vi "udpLoop.vi"(8 "error in (no error)":errorcluster) -> (0 "error out":errorcluster)   [LabVIEW 2015]
uses:
  Shared Libraries/CustomVIs/CustomVI.lvlib
panel:
  out "Connections Attempted":i32
  out "Remote Port":u16
  out "Remote Address":string
  in  "Local Interface":string="10.10.20.1"
  in  "Local Port":u16=50000
  out "IMUvalues":dbl[](array[numeric])
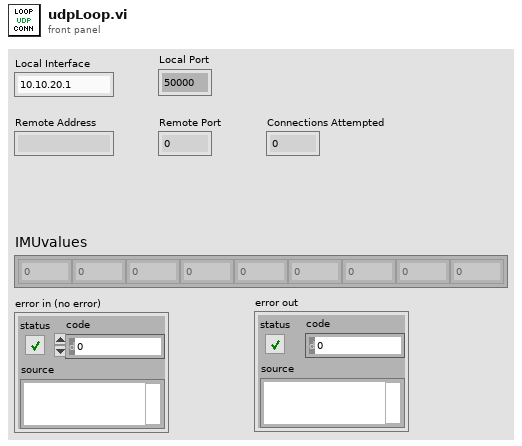
[diagram p1: front panel]
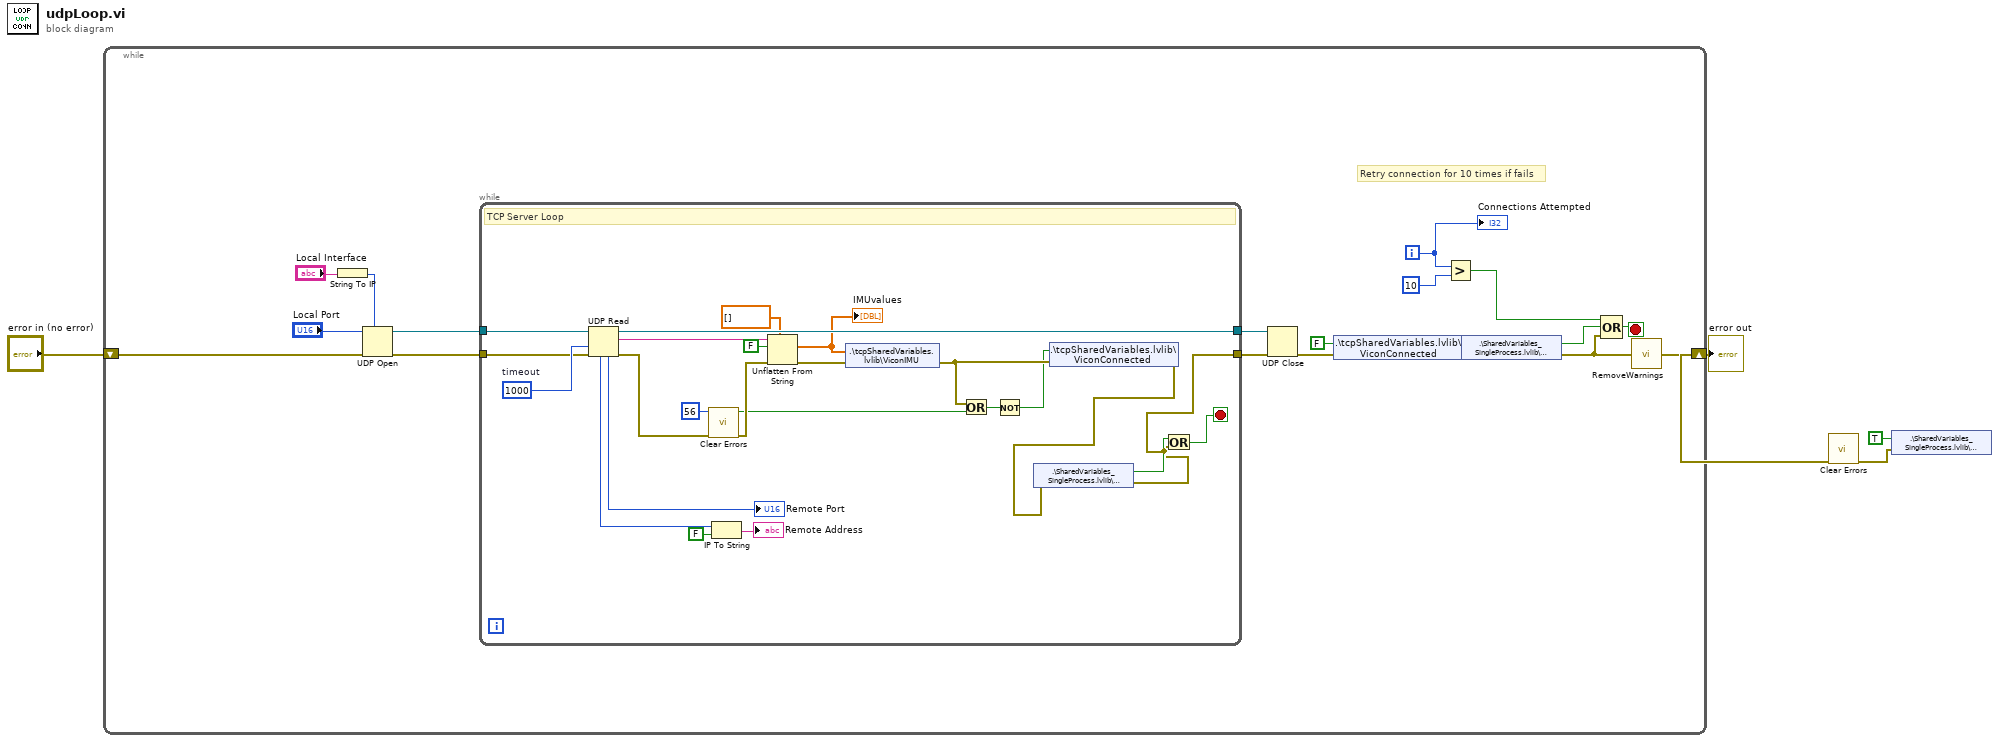
[diagram p0: block diagram]
diagram:
  n1 = while {
    shift-right: [w5] -> w1
    shift-left: "error in (no error)" -> [w17]
    i -> [w9]
    stop <- w14 stop-if-true
    # "Retry connection for 10 times if fails"
    n2 = String To IP(1:"Local Interface") -> (0:w21:u32)
    n3 = UDP Open(7:w21, 8:w17, 11:"Local Port") -> (port=w12:refnum<k16>, 0:w11:errorcluster)  [unwired: 2 in, 1 out]
    n4 = while {
      tunnel: [w27] -> w22
      tunnel: [w46] -> w10
      tunnel: w12 -> [w44]
      tunnel: w11 -> [w43]
      stop <- w28 stop-if-true
      w45 = 1000  # timeout
      # "TCP Server Loop"
      n5 = UDP Read(connection ID=w44, timeout ms (25000)=w45, 8:w43) -> (data out=w42:string, error out=w33:errorcluster, 3:w46:refnum<k16>, 4:→"Remote Port":u16, 6:w38:u32)  [unwired: 1 in]
      n6 = call <vilib>:"Clear Errors.vi"("error in (no error)"=w33, "specific error code to clear (0: all)"=56) -> ("error out"=w31:errorcluster, "specific error cleared?"=w26:bool)  [unwired: 4 in]
      n7 = IP To String(1:FALSE ("dot notation? (F)"), 2:w38) -> (0:→"Remote Address":string)
      n8 = Unflatten From String(type=dbl[] [] ("Waveform Graph 2"), binary string=w42, data includes array or string size? (T)=FALSE, error in (no error)=w31) -> (value=w39:dbl[], error out=w34:errorcluster)  [unwired: 1 in, 1 out]
      "IMUvalues" <- w39
      n9 = shared-variable ".\\tcpSharedVariables.lvlib\\ViconIMU"(w39, error in=w34) -> (error out=w25:errorcluster)
      n10 = Or(x=w25, y=w26) -> (x .or. y?=w24:bool)
      n11 = Not(x=w24) -> (.not. x?=w23:bool)
      n12 = shared-variable ".\\tcpSharedVariables.lvlib\\ViconConnected"(w23, error in=w25) -> (error out=w30:errorcluster)
      n13 = shared-variable ".\\SharedVariables_SingleProcess.lvlib\\GlobalStop"(error in=w30) -> (w29:bool, error out=w27:errorcluster)
      n14 = Or(x=w29, y=w27) -> (x .or. y?=w28:bool)
    }
    n15 = UDP Close(connection ID=w10, 8:w22) -> (error out=w19:errorcluster)  [unwired: 1 out]
    n16 = shared-variable ".\\tcpSharedVariables.lvlib\\ViconConnected"(FALSE ("Connected"), error in=w19) -> (error out=w16:errorcluster)
    n17 = Greater?(x=w9, y=10) -> (0:w7:bool)
    n18 = shared-variable ".\\SharedVariables_SingleProcess.lvlib\\GlobalStop"(error in=w16) -> (w15:bool, error out=w6:errorcluster)
    n19 = Compound Arithmetic op=OR(w7, w15, w6) -> (w14:bool)
    n20 = call "RemoveWarnings.vi"("error in (no error)"=w6) -> ("error out"=w5:errorcluster)
    "Connections Attempted" <- w9
  }
  "error out" <- w1
  n21 = call <vilib>:"Clear Errors.vi"("error in (no error)"=w1) -> ("error out"=w2:errorcluster)  [unwired: 5 in, 1 out]
  n22 = shared-variable ".\\SharedVariables_SingleProcess.lvlib\\GlobalStop"(TRUE ("GlobalStop"), error in=w2) -> ()  [unwired: 1 out]
